vi "Shift Picture Origin.vi"(8 "error in (no error)":errorcluster, 10 "Shift(0, 0)":T1, 11 "image data IN":T2) -> (0 "error out":errorcluster, 3 "image data OUT":T2)   [LabVIEW 2020]
doc: "<b> </b> <b> </b>\n©2013, Q Software Innovations, LLC.\n\nWritten in National Instruments LabVIEW™ 2013.\n\nAuthored by Quentin Alldredge\nQ@qsoftwareinnovations.com\nwww.qsoftwareinnovations.com\n\nAll rights reserved."
uses:
  <vilib>/picture/picture.llb/imagedata.ctl
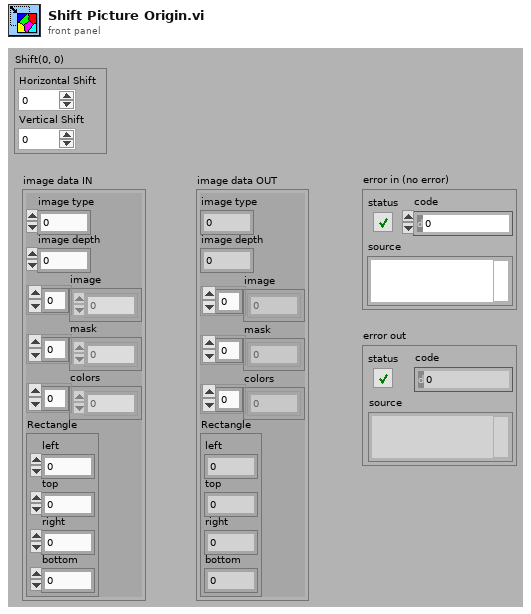
[diagram p1: front panel]
types:
  T1 = cluster{"Horizontal Shift":i16, "Vertical Shift":i16}
  T2 = typedef "imagedata.ctl" = cluster{"image type":i32, "image depth":i32, "image":u8[], "mask":u8[], "colors":u32[], "Rectangle":cluster{"left":i16, "top":i16, "right":i16, "bottom":i16}}
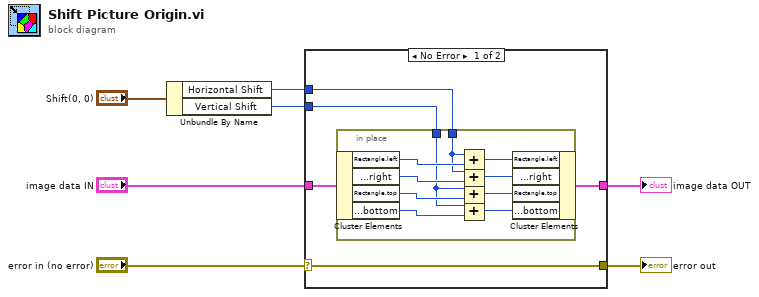
[diagram p0: block diagram]
diagram:
  n1 = Unbundle By Name("Shift(0, 0)") -> ("Horizontal Shift"=w2:i16, "Vertical Shift"=w1:i16)
  n2 = case shown="No Error" "error in (no error)" {
    selector: "error in (no error)" -> [w8 w23]
    tunnel: [w12 w24] -> w7
    tunnel: "image data IN" -> [w11 w24]
    tunnel: w2 -> [w10 _]
    tunnel: w1 -> [w9 _]
    tunnel: [w8 w23] -> w4
    frame No Error {
      n3 = in-place {
        in-place-border: w10 -> [w14]
        in-place-border: w9 -> [w13]
        n4 = in-place-cluster #1(w11) -> ("Rectangle.left"=w22:i16, "Rectangle.right"=w20:i16, "Rectangle.top"=w18:i16, "Rectangle.bottom"=w17:i16)
        n5 = Add(x=w14, y=w22) -> (x+y=w21:i16)
        n6 = Add(x=w14, y=w20) -> (x+y=w19:i16)
        n7 = Add(x=w13, y=w18) -> (x+y=w16:i16)
        n8 = Add(x=w13, y=w17) -> (x+y=w15:i16)
        n9 = in-place-cluster #1("Rectangle.left"=w21, "Rectangle.right"=w19, "Rectangle.top"=w16, "Rectangle.bottom"=w15) -> (w12:T2)
      }
    }
    frame Error {
    }
  }
  "image data OUT" <- w7
  "error out" <- w4
